vi "HRR-UartSend.vi"(8 "error in (no error)":errorcluster, 10 "Array":u8[][](array[numeric]), 11 "Refnum in":refnum<k20>) -> (0 "error out":errorcluster, 3 "Refnum out":refnum<k20>)   [LabVIEW 2019]
uses:
  <vilib>/Utility/error.llb/Error Cluster From Error Code.vi
  <vilib>/rvi/errors/niLvFpgaAdjustHostInterfaceError.vi
  <vilib>/rvi/interface/nirviMethod/nirviMethod.xnode
  <vilib>/FPGAPlugInAG/Dynamic/niLvFpga_WriteFifo_Dynamic.vi
  <vilib>/rvi/errors/niLvFpgaMergeErrorWithErrorCode.vi
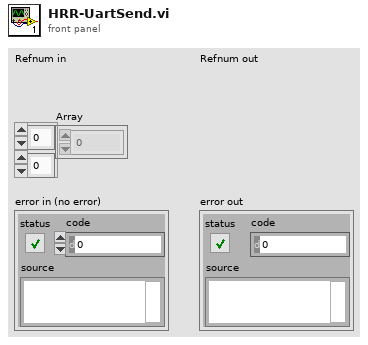
[diagram p1: front panel]
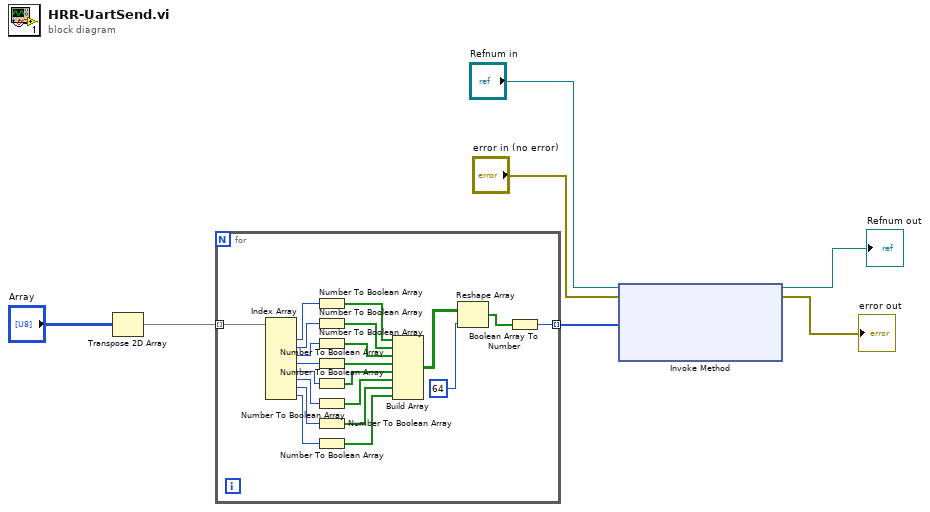
[diagram p0: block diagram]
diagram:
  n1 = Transpose 2D Array(2D array="Array") -> (transposed array=w1:u8[][])
  n2 = for {
    tunnel: w1 -> [w28] mode=indexing
    tunnel: [w8] -> w3 mode=indexing
    n3 = Index Array(array=w28) -> (element #1=w27:u8, element #2=w26:u8, element #3=w25:u8, element #4=w24:u8, element #5=w23:u8, element #6=w22:u8, element #7=w21:u8, element #8=w20:u8)  [unwired: 8 in]
    n4 = Number To Boolean Array(number=w27) -> (Boolean array=w19:bool[])
    n5 = Number To Boolean Array(number=w26) -> (Boolean array=w18:bool[])
    n6 = Number To Boolean Array(number=w25) -> (Boolean array=w17:bool[])
    n7 = Number To Boolean Array(number=w24) -> (Boolean array=w16:bool[])
    n8 = Number To Boolean Array(number=w23) -> (Boolean array=w15:bool[])
    n9 = Number To Boolean Array(number=w22) -> (Boolean array=w14:bool[])
    n10 = Number To Boolean Array(number=w21) -> (Boolean array=w13:bool[])
    n11 = Number To Boolean Array(number=w20) -> (Boolean array=w12:bool[])
    n12 = Build Array(w19, w18, w17, w16, w15, w14, w13, w12) -> (w11:bool[][])
    n13 = Reshape Array(w11, 64 ("dimension size")) -> (w9:bool[])
    n14 = Boolean Array To Number(Boolean array=w9) -> (number=w8:u64)
  }
  n15 = xnode "Invoke Method"("FPGA VI Reference In"="Refnum in", "error in"="error in (no error)", "Data"=w3) -> ("FPGA VI Reference Out"=→"Refnum out":refnum<k20>, "error out"=→"error out":errorcluster)  [unwired: 1 in, 1 out]
